vi "get_taskQueues.vi"(0 "HGF_ThreadPool_Reference":refnum<class "HGF_Reference.lvclass">, 3 "timeout in ms (-1)":i32=-1, 5 "error in (no error)":errorcluster) -> (11 "got object?":bool, 13 "autoIncrementLimit":i32=-1, 14 "dup HGF_ThreadPool_Reference":refnum<class "HGF_Reference.lvclass">, 15 "taskQueue out":refnum<queue>, 16 "timeoutTaskQueueOut":i32, 17 "taskQueue in":refnum<queue>, 18 "timeoutTaskQueueIn":i32, 19 "error out":errorcluster)   [LabVIEW 2014, in "HGF_BaseClasses.lvlib" / "HGF_ThreadPool.lvclass"]
doc: "Read taskQueue reference."
uses:
  HGF_ThreadPool.lvclass
  HGF_Reference/HGF_Reference.lvclass
  HGF_Auxiliary/HGF_Auxiliary.lvlib
  HGF_ThreadTask/HGF_ThreadTask.lvclass
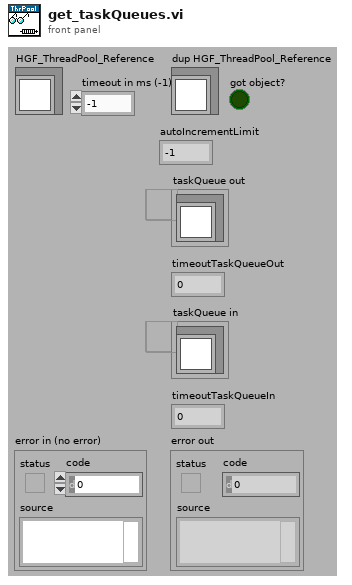
[diagram p1: front panel]
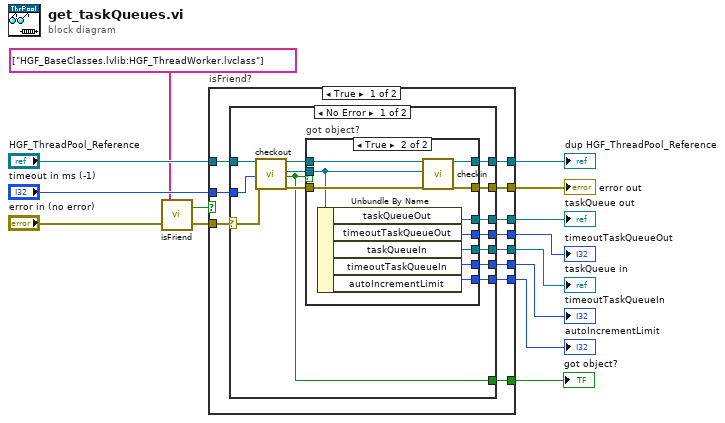
[diagram p0: block diagram]
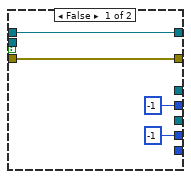
[diagram p2: hidden frame]
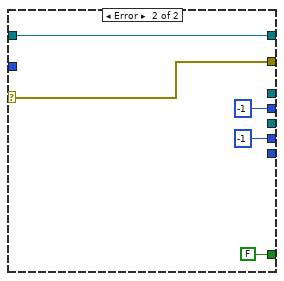
[diagram p3: hidden frame]
diagram:
  n1 = call "isFriend.vi"("error in (no error)"="error in (no error)", "Friends"=string[] ["HGF_BaseClasses.lvlib:HGF_ThreadWorker.lvclass"]) -> ("error out"=w3:errorcluster, "isFriend?"=w2:bool)
  n2 = case "isFriend?" shown="True" w2 {
    tunnel: w3 -> [w25 w59]
    tunnel: [w24 w59] -> w14
    tunnel: "HGF_ThreadPool_Reference" -> [w23 w60]
    tunnel: [w22 w60] -> w12
    tunnel: [w21 _] -> w11
    tunnel: [w20 _] -> w10
    tunnel: [w19 _] -> w9
    tunnel: [w18 _] -> w8
    tunnel: "timeout in ms (-1)" -> [w17 _]
    tunnel: [w16 _] -> w6
    tunnel: [w15 _] -> w1
    frame True {
      n3 = case shown="No Error" w25 {
        selector: w25 -> [w34 w57]
        tunnel: [w29 w57] -> w24
        tunnel: [w31 w58] -> w22
        tunnel: w23 -> [w35 w58]
        tunnel: [w39 _] -> w21
        tunnel: [w38 _] -> w20
        tunnel: [w37 -1 ("timeoutTaskQueueOut")] -> w19
        tunnel: [w36 -1 ("timeoutTaskQueueIn")] -> w18
        tunnel: w17 -> [w28 _]
        tunnel: [w27 FALSE ("got object?")] -> w16
        tunnel: [w26 _] -> w15
        frame No Error {
          n4 = call "checkout.vi"("HGF_ThreadPool_Reference"=w35, "timeout in ms (-1)"=w28, "error in (no error)"=w34) -> ("dup HGF_ThreadPool_Reference"=w32:refnum<class "HGF_Reference.lvclass">, "HGF_ThreadPool"=w33:refnum<class "HGF_ThreadPool.lvclass">, "got object?"=w27:bool, "error out"=w30:errorcluster)  [unwired: 13 out]
          n5 = case "got object?" shown="True" w27 {
            tunnel: [_ w53] -> w39
            tunnel: [_ w52] -> w38
            tunnel: [-1 ("timeoutTaskQueueOut") w51] -> w37
            tunnel: [-1 ("timeoutTaskQueueIn") w50] -> w36
            tunnel: w33 -> [_ w45]
            tunnel: w32 -> [w43 w49]
            tunnel: w30 -> [w42 w48]
            tunnel: [w43 w47] -> w31
            tunnel: [w42 w46] -> w29
            tunnel: [_ w44] -> w26
            frame False {
            }
            frame True {
              n6 = Unbundle By Name(w45) -> ("taskQueueOut"=w52:refnum<queue>, "timeoutTaskQueueOut"=w51:i32, "taskQueueIn"=w53:refnum<queue>, "timeoutTaskQueueIn"=w50:i32, "autoIncrementLimit"=w44:i32)
              n7 = call "checkin.vi"("HGF_Reference"=w49, "Object"=w45, "error in (no error)"=w48) -> ("dup HGF_Reference"=w47:refnum<class "HGF_Reference.lvclass">, "error out"=w46:errorcluster)  [unwired: 1 in, 14 out]
            }
          }
        }
        frame Error {
        }
      }
    }
    frame False {
    }
  }
  "error out" <- w14
  "dup HGF_ThreadPool_Reference" <- w12
  "taskQueue in" <- w11
  "taskQueue out" <- w10
  "timeoutTaskQueueOut" <- w9
  "timeoutTaskQueueIn" <- w8
  "got object?" <- w6
  "autoIncrementLimit" <- w1
